vi "MGCC_Commun_PollIndex.vi"(11 "Analog Input Indexes":u16[](array[numeric])) -> (3 "Poll":T1[](array[typedef]))   [LabVIEW 2016]
uses:
  <vilib>/DNP3/DNP3_Master/Start Stop.ctl
  <vilib>/DNP3/DNP3_Master.lvlib
panel:
  out "stop":i32
  out "Numeric":i32
  out "start":u16
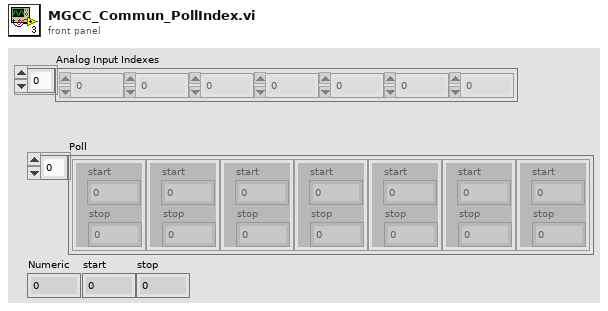
[diagram p1: front panel]
types:
  T1 = typedef "DNP3_Master.lvlib/Start Stop.ctl" = cluster{"start":u16, "stop":u16}
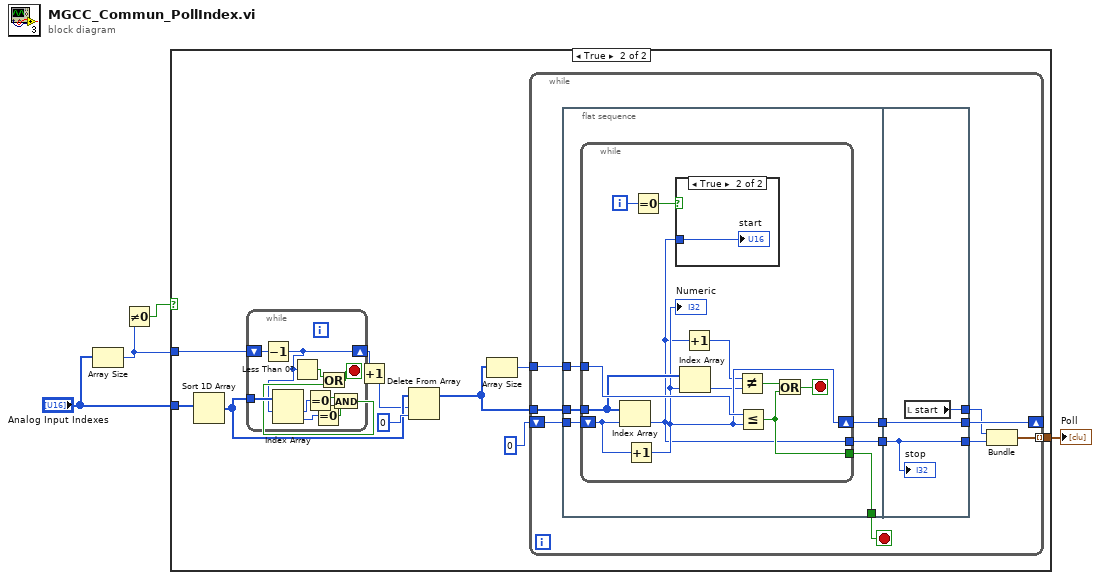
[diagram p0: block diagram]
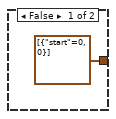
[diagram p2: hidden frame]
diagram:
  n1 = Array Size(array="Analog Input Indexes") -> (size(s)=w1:i32)
  n2 = Not Equal To 0?(x=w1) -> (x != 0?=w3:bool)
  n3 = case shown="True" w3 {
    tunnel: [cluster{"start":u16, u16}[] [{"start"=0, 0}] w15] -> w4
    tunnel: "Analog Input Indexes" -> [_ w10]
    tunnel: w1 -> [_ w9]
    frame False {
    }
    frame True {
      n4 = Sort 1D Array(array=w10) -> (sorted array=w8:u16[])
      n5 = while {
        shift-right: [w16] -> w7
        shift-left: w9 -> [w18]
        tunnel: w8 -> [w25]
        stop <- w24 stop-if-true
        n6 = Decrement(x=w18) -> (x-1=w16:i32)
        n7 = Index Array(array=w25, index #1=w16) -> (element #1=w23:u16, element #2=w22:u16)  [unwired: 1 in]
        n8 = Less Than 0?(x=w16) -> (x < 0?=w17:bool)
        n9 = Equal To 0?(x=w23) -> (x = 0?=w21:bool)
        n10 = Equal To 0?(x=w22) -> (x = 0?=w20:bool)
        n11 = And(x=w21, y=w20) -> (x .and. y?=w19:bool)
        n12 = Or(x=w17, y=w19) -> (x .or. y?=w24:bool)
      }
      n13 = Increment(x=w7) -> (x+1=w6:i32)
      n14 = Delete From Array(array=w8, length=w6, index=0) -> (array with subset deleted=w11:u16[])  [unwired: 1 out]
      n15 = Array Size(array=w11) -> (size(s)=w13:i32)
      n16 = while {
        tunnel: w11 -> [w34]
        tunnel: w13 -> [w35]
        shift-right: [w33] -> _
        shift-left: 0 -> [w32]
        tunnel: [w31] -> w15 mode=indexing
        stop <- w28 stop-if-true
        n17 = flat-sequence {
          tunnel: w35 -> [w41]
          tunnel: w34 -> [w40]
          tunnel: w32 -> [w38]
          tunnel: [w39] -> w30
          tunnel: [w37] -> w28
          tunnel: [w36] -> w27
          tunnel: [w57] -> w33
          tunnel: w30 -> [w57]
          tunnel: [w56] -> w29
          tunnel: w27 -> [w55]
          tunnel: [w55] -> w26
          frame #0 {
            n18 = while {
              tunnel: w41 -> [w53]
              tunnel: w40 -> [w46]
              shift-right: [w45] -> w39
              shift-left: w38 -> [w52]
              tunnel: [w47] -> w37
              tunnel: [w42] -> w36
              i -> [w49]
              stop <- w51 stop-if-true
              n19 = Index Array(array=w46, index=w52) -> (element=w42:u16)
              n20 = Increment(x=w52) -> (x+1=w45:i32)
              "Numeric" <- w45
              n21 = Equal To 0?(x=w49) -> (x = 0?=w48:bool)
              n22 = case shown="True" w48 {
                tunnel: w42 -> [_ w54]
                frame False {
                }
                frame True {
                  "start" <- w54
                }
              }
              n23 = Index Array(array=w46, index=w45) -> (element=w43:u16)
              n24 = Increment(x=w42) -> (x+1=w44:u16)
              n25 = Not Equal?(x=w44, y=w43) -> (x != y?=w50:bool)
              n26 = Less Or Equal?(x=w53, y=w45) -> (x <= y?=w47:bool)
              n27 = Or(x=w50, y=w47) -> (x .or. y?=w51:bool)
            }
          }
          frame #1 {
            n28 = local read "start"() -> (w56:u16)
            "stop" <- w55
          }
        }
        n29 = Bundle("start"=w29, w26) -> (w31:cluster{"start":u16, u16})  [unwired: 1 in]
      }
    }
  }
  "Poll" <- w4
